vi "Find or Create Month Folder.vi"() -> (3 "Month Folder":path)   [LabVIEW 2017]
uses:
  ABB global.vi
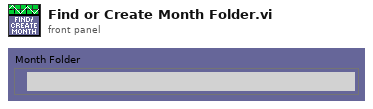
[diagram p1: front panel]
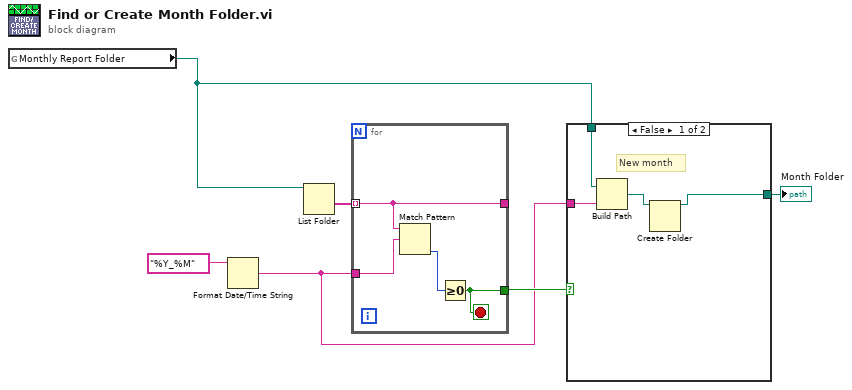
[diagram p0: block diagram]
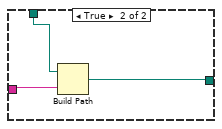
[diagram p2: hidden frame]
diagram:
  n1 = global read "ABB global.vi" "Monthly Report Folder"() -> (w3:path)
  n2 = Format Date/Time String(time format string (%c)="%Y_%M") -> (date/time string=w1:string)  [unwired: 2 in]
  n3 = List Folder(path=w3) -> (folder names=w5:string[])  [unwired: 3 in, 3 out]
  n4 = for {
    tunnel: w5 -> [w8] mode=indexing
    tunnel: w1 -> [w10]
    tunnel: [w8] -> _
    tunnel: [w7] -> w4
    stop <- w7 stop-if-true
    n5 = Match Pattern(string=w8, regular expression=w10) -> (offset past match=w9:i32)  [unwired: 1 in, 3 out]
    n6 = Greater Or Equal To 0?(x=w9) -> (x >= 0?=w7:bool)
  }
  n7 = case shown="False" w4 {
    tunnel: w1 -> [w13 w16]
    tunnel: w3 -> [w14 w17]
    tunnel: [w11 w15] -> w2
    frame False {
      # "New month"
      n8 = Build Path(base path=w14, name or relative path=w13) -> (appended path=w12:path)
      n9 = Create Folder(path (use dialog)=w12) -> (created path=w11:path)  [unwired: 2 in, 2 out]
    }
    frame True {
      n10 = Build Path(base path=w17, name or relative path=w16) -> (appended path=w15:path)
    }
  }
  "Month Folder" <- w2
